vi "AVI Video Save.vi"(5 "Frame Size":u32, 6 "Channel":T1, 7 "AVI mode":T6, 8 "error in (no error)":errorcluster, 9 "AVI cluster":T2, 10 "PMT is ON?":bool, 11 "Image Pixels":i16[][](array[numeric])) -> (0 "error out":errorcluster, 2 "New split file has just been initialised":bool)   [LabVIEW 2017]
uses:
  Typedefs/AVI implementation enum.ctl
  Typedefs/AVI Refs cluster.ctl
  <vilib>/vision/Avi.llb/IMAQ AVI2 Refnum.ctl
  <vilib>/vision/Image Controls.llb/IMAQ Image.ctl
  <vilib>/vision/Avi1.llb/AviRefnum.ctl
  Typedefs/Channel Selector.ctl
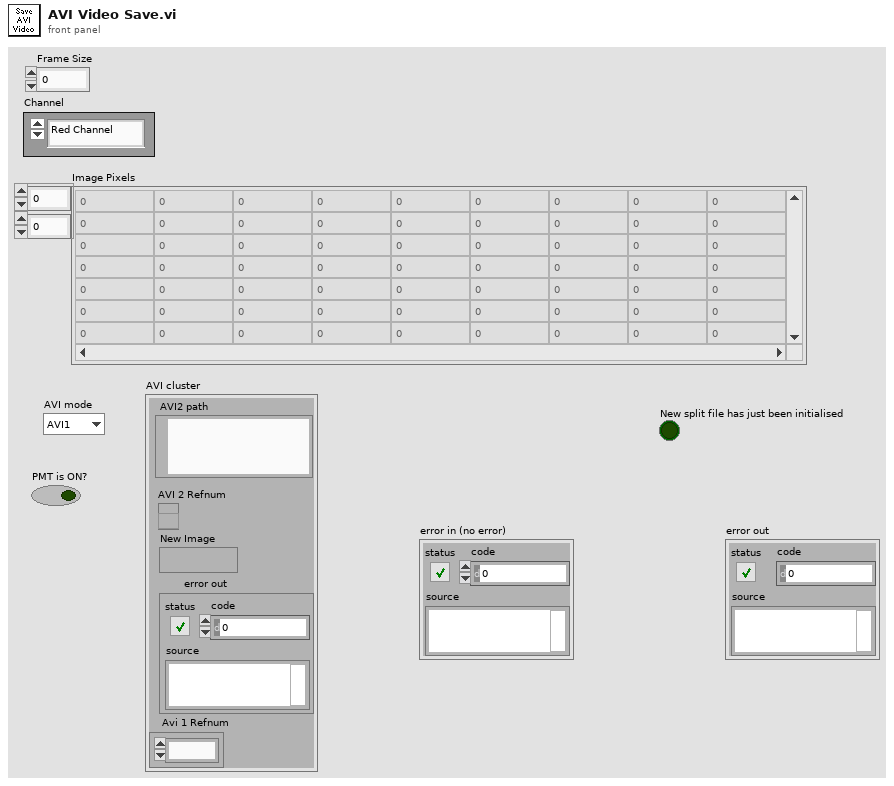
[diagram p1: front panel]
types:
  T1 = typedef "Channel Selector.ctl" = enum16{"Red Channel", "Green Channel", "Blended"}
  T2 = typedef "AVI Refs cluster.ctl" = cluster{"AVI2 path":path, "AVI 2 Refnum":T3, "New Image":T4, "error out":errorcluster, "Avi 1 Refnum":T5}
  T3 = typedef "IMAQ AVI2 Refnum.ctl" = refnum<k20>
  T4 = typedef "IMAQ Image.ctl" = refnum<image>
  T5 = typedef "AviRefnum.ctl" = refnum<k1>
  T6 = typedef "AVI implementation enum.ctl" = enum16{"AVI1", "AVI2"}
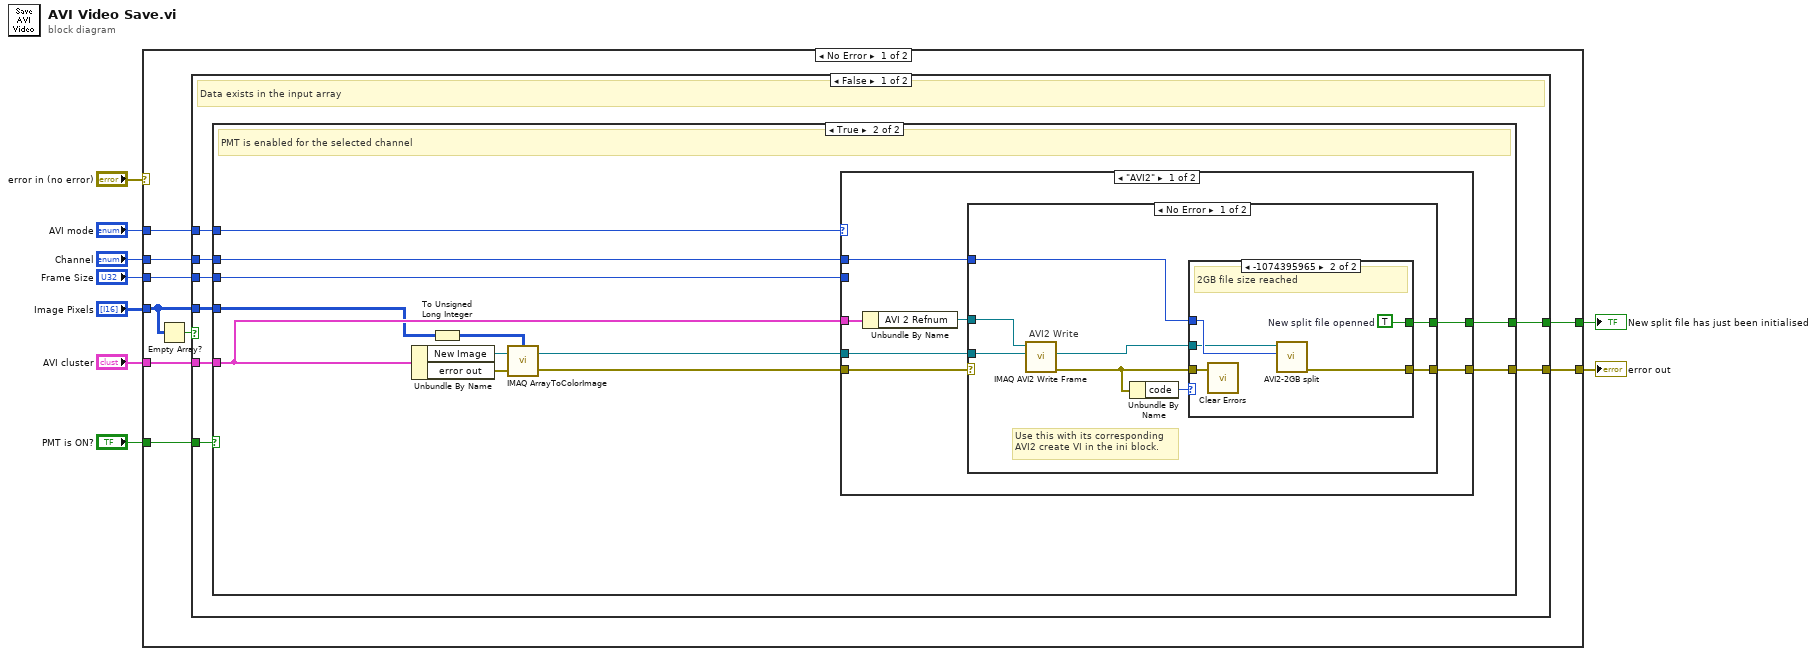
[diagram p0: block diagram]
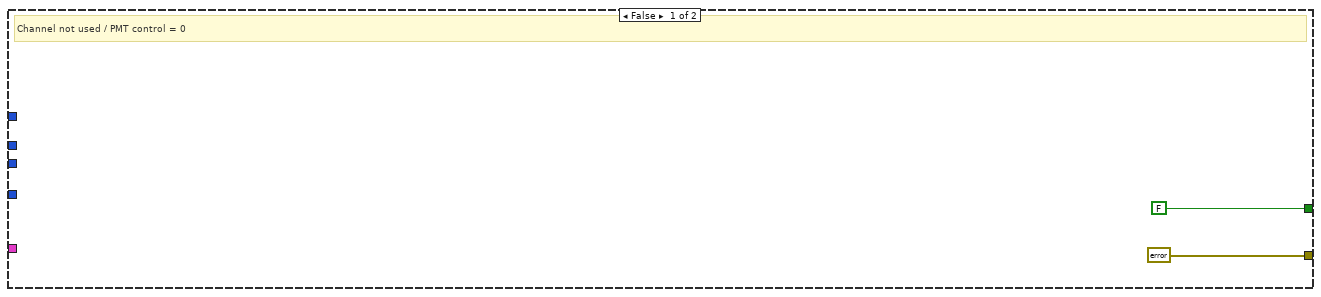
[diagram p2: hidden frame]
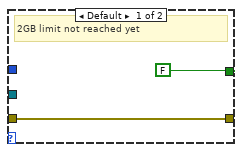
[diagram p3: hidden frame]
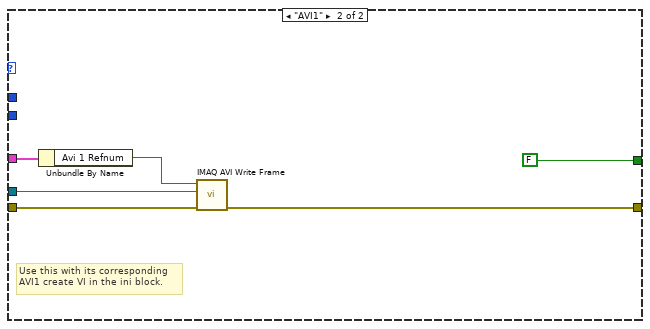
[diagram p5: hidden frame]
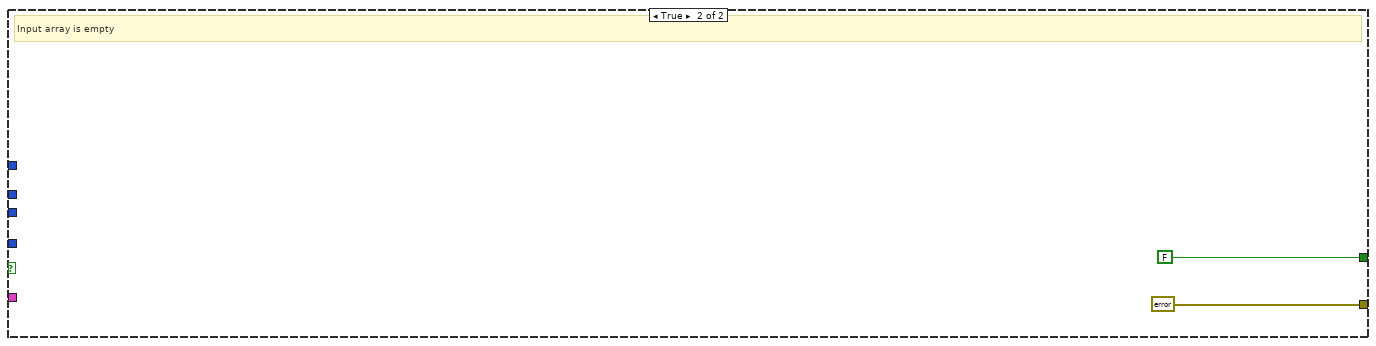
[diagram p6: hidden frame]
diagram:
  n1 = case shown="No Error" "error in (no error)" {
    tunnel: [w18 _] -> w7
    tunnel: "Image Pixels" -> [w10 _]
    tunnel: "AVI mode" -> [w17 _]
    tunnel: "AVI cluster" -> [w16 _]
    tunnel: "PMT is ON?" -> [w15 _]
    tunnel: "Channel" -> [w14 _]
    tunnel: [w13 _] -> w2
    tunnel: "Frame Size" -> [w12 _]
    frame No Error {
      n2 = Empty Array?(array=w10) -> (empty?=w11:bool)
      n3 = case shown="False" w11 {
        tunnel: w10 -> [w26 _]
        tunnel: [w25 errorcluster {"status"=FALSE, "code"=0, "source"=""} ("error out")] -> w18
        tunnel: w17 -> [w24 _]
        tunnel: w16 -> [w23 _]
        tunnel: w15 -> [w22 _]
        tunnel: w14 -> [w21 _]
        tunnel: [w20 FALSE] -> w13
        tunnel: w12 -> [w19 _]
        frame False {
          # "Data exists in the input array"
          n4 = case shown="True" w22 {
            tunnel: w26 -> [_ w33]
            tunnel: w23 -> [_ w36]
            tunnel: [errorcluster {"status"=FALSE, "code"=0, "source"=""} ("error out") w38] -> w25
            tunnel: w24 -> [_ w37]
            tunnel: w21 -> [_ w32]
            tunnel: [FALSE w35] -> w20
            tunnel: w19 -> [_ w34]
            frame False {
              # "Channel not used / PMT control = 0"
            }
            frame True {
              # "PMT is enabled for the selected channel"
              n5 = Unbundle By Name(w36) -> ("New Image"=w31:T4, "error out"=w30:errorcluster)
              n6 = To Unsigned Long Integer(number=w33) -> (unsigned 32bit integer=w29:u32[][])
              n7 = call "IMAQ ArrayToColorImage"("Image Pixels (U32)"=w29, "Image"=w31, "error in (no error)"=w30) -> ("Image Out"=w39:T4, "error out"=w40:errorcluster)  [unwired: 1 in, 1 out]
              n8 = case shown="\"AVI2\"" w37 {
                tunnel: w40 -> [w47 w69]
                tunnel: w39 -> [w46 w68]
                tunnel: [w44 w67] -> w38
                tunnel: w36 -> [w45 w65]
                tunnel: w32 -> [w43 _]
                tunnel: [w42 FALSE] -> w35
                tunnel: w34 -> [_ _]
                frame "AVI2" {
                  n9 = Unbundle By Name(w45) -> ("AVI 2 Refnum"=w41:T3)
                  n10 = case shown="No Error" w47 {
                    selector: w47 -> [_ w63]
                    tunnel: w46 -> [w51 _]
                    tunnel: [w55 w63] -> w44
                    tunnel: w43 -> [w54 _]
                    tunnel: w41 -> [w53 _]
                    tunnel: [w49 _] -> w42
                    frame No Error {
                      # "AVI2 Write"
                      # "Use this with its corresponding\nAVI2 create VI in the ini block."
                      n11 = call "IMAQ AVI2 Write Frame"("Image"=w51, "AVI Refnum"=w53) -> ("error out"=w52:errorcluster, "Image Out (duplicate)"=w48:T4)  [unwired: 7 in, 1 out]
                      n12 = Unbundle By Name(w52) -> ("code"=w50:i32)
                      n13 = case shown="-1074395965" w50 {
                        tunnel: [w57 w60] -> w55
                        tunnel: w54 -> [_ w62]
                        tunnel: w52 -> [w57 w61]
                        tunnel: [FALSE w58] -> w49
                        tunnel: w48 -> [_ w59]
                        frame Default {
                          # "2GB limit not reached yet"
                        }
                        frame -1074395965 {
                          w58 = TRUE  # New split file openned
                          # "2GB file size reached"
                          n14 = call <vilib>:"Clear Errors.vi"("error in (no error)"=w61) -> ()  [unwired: 5 in, 2 out]
                          n15 = call "AVI2-2GB split.vi"("Channel"=w62, "Timelapse frame that couldn't be written"=w59) -> ("error out"=w60:errorcluster)  [unwired: 9 in]
                        }
                      }
                    }
                    frame Error {
                    }
                  }
                }
                frame "AVI1" {
                  # "Use this with its corresponding\nAVI1 create VI in the ini block."
                  n16 = Unbundle By Name(w65) -> ("Avi 1 Refnum"=w66:T5)
                  n17 = call "IMAQ AVI Write Frame"("error in (no error)"=w69, "Image"=w68, "Avi Refnum"=w66) -> ("error out"=w67:errorcluster)  [unwired: 7 in, 1 out]
                }
              }
            }
          }
        }
        frame True {
          # "Input array is empty"
        }
      }
    }
    frame Error {
    }
  }
  "error out" <- w7
  "New split file has just been initialised" <- w2
